vi "MSScript_Transform_UInt.vi"(5 "upper limit":u64=18446744073709551615, 7 "lower limit":u64, 11 "string in":string) -> (1 "Is a variable ?":bool, 2 "Value Error?":bool, 3 "Value Output":u64)   [LabVIEW 2018, in "MSScript.lvclass"]
uses:
  MSScript.lvclass
  <vilib>/regexp/Match Regular Expression.xnode
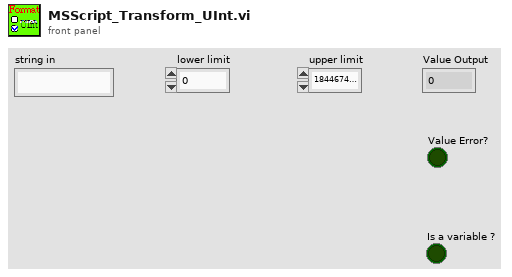
[diagram p1: front panel]
types:
  T1 = enum16{"Scalar", "ScalarArray", "Var", "VarArray", "Error"}
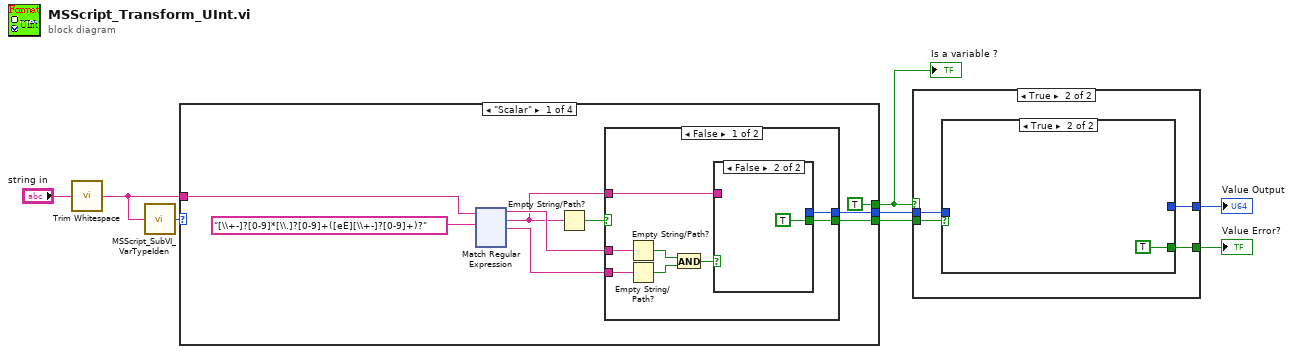
[diagram p0: block diagram]
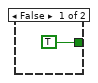
[diagram p2: hidden frame]
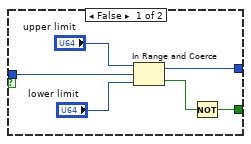
[diagram p3: hidden frame]
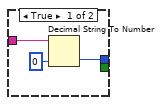
[diagram p4: hidden frame]
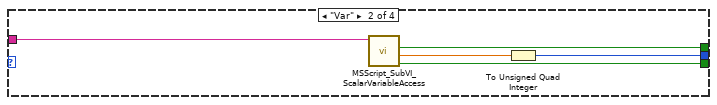
[diagram p6: hidden frame]
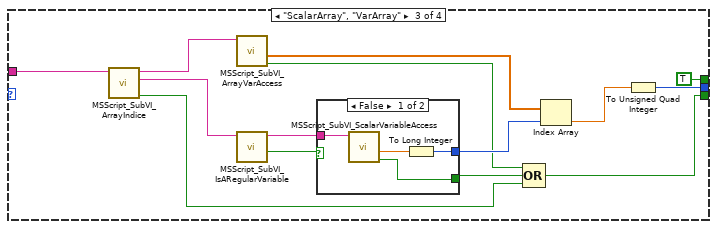
[diagram p7: hidden frame]
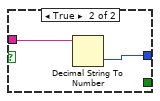
[diagram p8: hidden frame]
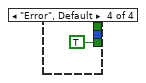
[diagram p9: hidden frame]
diagram:
  n1 = call <vilib>:"Trim Whitespace.vi"("string"="string in") -> ("trimmed string"=w2:string)  [unwired: 1 in]
  n2 = call "MSScript_SubVI_VarTypeIden.vi"("Var in"=w2) -> ("Type"=w1:T1)
  n3 = case shown="\"Scalar\"" w1 {
    tunnel: [w13 w145 w152 TRUE ("Value Error?")] -> w5
    tunnel: [w12 w147 w150 _] -> w7
    tunnel: w2 -> [w10 w149 w154 _]
    tunnel: [TRUE ("Is a variable ?") w146 TRUE ("Is a variable ?") _] -> w6
    frame "Scalar" {
      n4 = xnode "Match Regular Expression"("input string"=w10, "regular expression"="[\\+-]?[0-9]*[\\.]?[0-9]+([eE][\\+-]?[0-9]+)?") -> ("before match"=w16:string, "whole match"=w14:string, "after match"=w15:string)  [unwired: 4 in, 2 out]
      n5 = Empty String/Path?(string/path=w14) -> (empty?=w17:bool)
      n6 = case shown="False" w17 {
        selector: w17 -> [_ w144]
        tunnel: [w134 w144] -> w13
        tunnel: w16 -> [w136 _]
        tunnel: w15 -> [w137 _]
        tunnel: w14 -> [w133 _]
        tunnel: [w132 _] -> w12
        frame False {
          n7 = Empty String/Path?(string/path=w136) -> (empty?=w138:bool)
          n8 = Empty String/Path?(string/path=w137) -> (empty?=w139:bool)
          n9 = And(x=w138, y=w139) -> (x .and. y?=w135:bool)
          n10 = case shown="False" w135 {
            tunnel: [_ TRUE] -> w134
            tunnel: w133 -> [w142 _]
            tunnel: [w140 _] -> w132
            frame True {
              n11 = Decimal String To Number(string=w142, default (0L)=u64 0 ("default (0 I32)")) -> (number=w140:u64)  [unwired: 1 in, 1 out]
            }
            frame False {
            }
          }
        }
        frame True {
        }
      }
    }
    frame "Var" {
      n12 = call "MSScript_SubVI_ScalarVariableAccess.vi"("VarName"=w149) -> ("Value Error?"=w145:bool, "OutputValue"=w148:ext, "Is a variable ?"=w146:bool)  [unwired: 6 in]
      n13 = To Unsigned Quad Integer(1:w148) -> (0:w147:u64)
    }
    frame "ScalarArray", "VarArray" {
      n14 = call "MSScript_SubVI_ArrayIndice.vi"("@name[x:y|z]"=w154) -> ("Index no found"=w155:bool, "Indice string"=w162:string, "@name"=w163:string)  [unwired: 6 in]
      n15 = call "MSScript_SubVI_ArrayVarAccess.vi"("VarName"=w163) -> ("Value Error?"=w156:bool, "ArrayVariable out"=w159:ext[])  [unwired: 6 in, 1 out]
      n16 = call "MSScript_SubVI_IsARegularVariable.vi"("VarString in"=w162) -> ("Variable simbol no found"=w161:bool, "VarString out"=w160:string)  [unwired: 6 in, 1 out]
      n17 = case shown="False" w161 {
        tunnel: w160 -> [w167 w169]
        tunnel: [w165 w168] -> w158
        tunnel: [w164 _] -> w157
        frame False {
          n18 = call "MSScript_SubVI_ScalarVariableAccess.vi"("VarName"=w167) -> ("Value Error?"=w164:bool, "OutputValue"=w166:ext)  [unwired: 6 in, 1 out]
          n19 = To Long Integer(number=w166) -> (32bit integer=w165:i32)
        }
        frame True {
          n20 = Decimal String To Number(string=w169) -> (number=w168:i32)  [unwired: 2 in, 1 out]
        }
      }
      n21 = Compound Arithmetic op=OR(w156, w157, w155) -> (w152:bool)
      n22 = Index Array(array=w159, index=w158) -> (element=w151:ext)
      n23 = To Unsigned Quad Integer(1:w151) -> (0:w150:u64)
    }
    frame "Error", Default {
    }
  }
  "Is a variable ?" <- w6
  n24 = case shown="True" w6 {
    tunnel: w5 -> [_ w175]
    tunnel: w7 -> [_ w173]
    tunnel: [TRUE w174] -> w3
    tunnel: [_ w172] -> w4
    frame False {
    }
    frame True {
      n25 = case shown="True" w175 {
        tunnel: [w179 TRUE] -> w174
        tunnel: w173 -> [w176 _]
        tunnel: [w181 _] -> w172
        frame False {
          n26 = In Range and Coerce(upper limit="upper limit", x=w176, lower limit="lower limit") -> (coerced(x)=w181:u64, In Range?=w180:bool)
          n27 = Not(x=w180) -> (.not. x?=w179:bool)
        }
        frame True {
        }
      }
    }
  }
  "Value Error?" <- w3
  "Value Output" <- w4
